vi "CLAD-2 scratch.vi"() -> ()   [LabVIEW 2013]
panel:
  out "Numeric":dbl
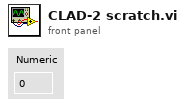
[diagram p1: front panel]
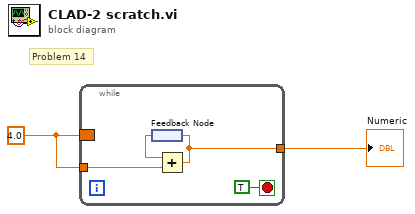
[diagram p0: block diagram]
diagram:
  w1 = 4.0
  # "Problem 14"
  n1 = while {
    tunnel: w1 -> [w5]
    tunnel: [w4] -> w2
    border: w1 -> [_]
    stop <- TRUE stop-if-true
    n2 = feedback #1() -> (w6:dbl)
    n3 = Add(x=w6, y=w5) -> (x+y=w4:dbl)
    n4 = feedback-in #1(w4) -> ()
  }
  "Numeric" <- w2
